vi "parse_sim_ini.vi"(11 "Parent path":path) -> (3 "SIM INI":T1)   [LabVIEW 2015]
uses:
  SIM INI.ctl
  <vilib>/Utility/config.llb/Read Key (Double).vi
  <vilib>/Utility/config.llb/NI_LVConfig.lvlib
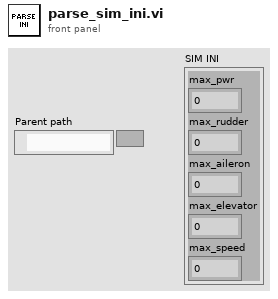
[diagram p1: front panel]
types:
  T1 = typedef "SIM INI.ctl" = cluster{"max_pwr":dbl, "max_rudder":dbl, "max_aileron":dbl, "max_elevator":dbl, "max_speed":dbl}
  T2 = typedef "NI_LVConfig.lvlib/Config Data RefNum.ctl" = refnum<k1>
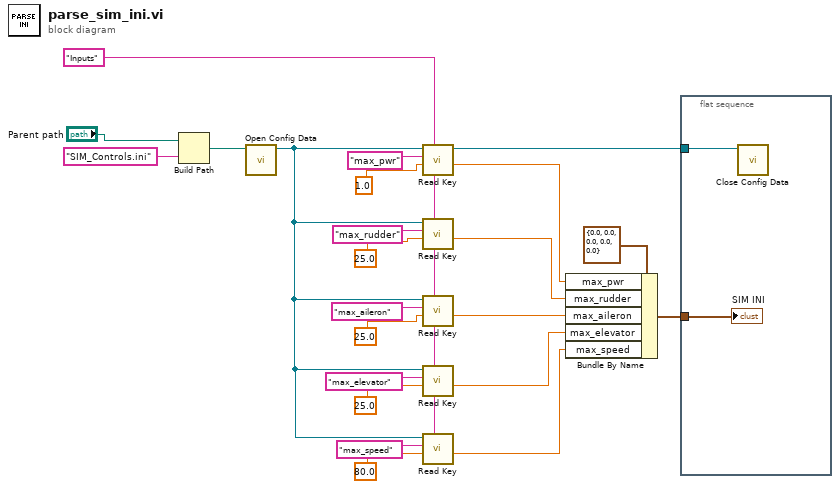
[diagram p0: block diagram]
diagram:
  w14 = "Inputs" ("section")
  n1 = Build Path(base path="Parent path", name or relative path="SIM_Controls.ini") -> (appended path=w20:path)
  n2 = call <vilib>:"Open Config Data.vi"("configuration file path"=w20) -> ("refnum"=w15:T2)  [unwired: 8 in, 2 out]
  n3 = call-poly <vilib>:"Read Key.vi"("section"=w14, "default value"=1.0, "key"="max_pwr", "refnum"=w15) -> ("value"=w12:dbl, "refnum out"=w7:T2)  [unwired: 4 in, 2 out]
  n4 = call-poly <vilib>:"Read Key.vi"("section"=w14, "default value"=25.0, "key"="max_rudder", "refnum"=w15) -> ("value"=w11:dbl)  [unwired: 4 in, 3 out]
  n5 = call-poly <vilib>:"Read Key.vi"("section"=w14, "default value"=25.0, "key"="max_aileron", "refnum"=w15) -> ("value"=w10:dbl)  [unwired: 4 in, 3 out]
  n6 = call-poly <vilib>:"Read Key.vi"("section"=w14, "default value"=25.0, "key"="max_elevator", "refnum"=w15) -> ("value"=w9:dbl)  [unwired: 4 in, 3 out]
  n7 = call-poly <vilib>:"Read Key.vi"("section"=w14, "default value"=80.0, "key"="max_speed", "refnum"=w15) -> ("value"=w8:dbl)  [unwired: 4 in, 3 out]
  n8 = Bundle By Name(cluster=T1 {"max_pwr"=0.0, "max_rudder"=0.0, "max_aileron"=0.0, "max_elevator"=0.0, "max_speed"=0.0}, "max_pwr"=w12, "max_rudder"=w11, "max_aileron"=w10, "max_elevator"=w9, "max_speed"=w8) -> (w6:T1)
  n9 = flat-sequence {
    tunnel: w7 -> [w25]
    tunnel: w6 -> [w24]
    frame #0 {
      n10 = call <vilib>:"Close Config Data.vi"("refnum"=w25) -> ()  [unwired: 9 in, 2 out]
      "SIM INI" <- w24
    }
  }
